vi "ContextHelp_Memory.vi"(0 "PopUpTaskEvent":T1, 1 "State":bool, 5 "error in (no error)":errorcluster, 6 "Actio(GetStatus)n":T2(ring)=enum."GetStatus") -> (14 "PopUpTaskEventOut":T1, 15 "Open":bool, 16 "DialogCaller":bool, 17 "DialogRef":refnum<vi>, 18 "ToolHelp":bool, 19 "error out":errorcluster)   [LabVIEW 2016]
uses:
  <resource>/Framework/Providers/Open_GDS/UML/ContextHelp/ContextHelp_EventType.ctl
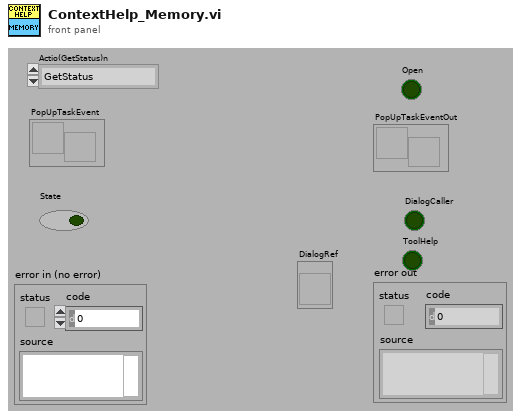
[diagram p1: front panel]
types:
  T1 = typedef "ContextHelp_EventType.ctl" = refnum<user-event>
  T2 = enum16{"SetPopUpEventTask", "GetStatus", "SetOpenState", "SetDialogCaller", "SetToolHelp"}
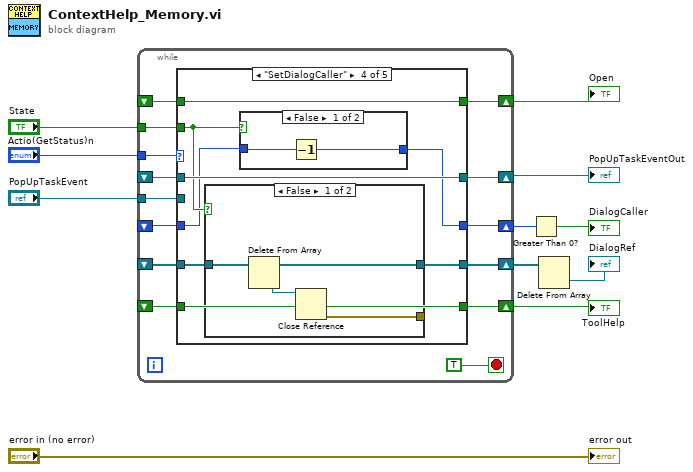
[diagram p0: block diagram]
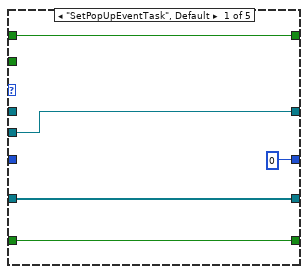
[diagram p2: hidden frame]
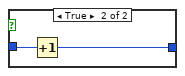
[diagram p5: hidden frame]
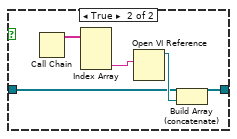
[diagram p6: hidden frame]
diagram:
  n1 = while {
    tunnel: "Actio(GetStatus)n" -> [w25]
    shift-right: [w23] -> w9
    shift-left: _ -> [w24]
    tunnel: "State" -> [w22]
    shift-right: [w21] -> w6
    shift-left: _ -> [w19]
    tunnel: "PopUpTaskEvent" -> [w20]
    shift-right: [w17] -> w4
    shift-left: _ -> [w16]
    shift-right: [w15] -> w2
    shift-left: _ -> [w14]
    shift-right: [w13] -> w5
    shift-left: _ -> [w12]
    stop <- TRUE stop-if-true
    n2 = case shown="\"SetDialogCaller\"" w25 {
      tunnel: w24 -> [w30 _ w36 w47 w66]
      tunnel: [w30 w35 w36 w47 w66] -> w23
      tunnel: w22 -> [_ w35 w37 w43 _]
      tunnel: [w29 w34 w40 w48 w65] -> w21
      tunnel: w20 -> [w29 _ _ _ _]
      tunnel: w19 -> [_ w34 w40 w48 w65]
      tunnel: [0 w33 w39 w41 w64] -> w17
      tunnel: w16 -> [_ w33 w39 w42 w64]
      tunnel: [w28 w32 w38 w46 w63] -> w15
      tunnel: w14 -> [w28 w32 w38 w45 w63]
      tunnel: [w27 w31 w37 w44 w62] -> w13
      tunnel: w12 -> [w27 w31 _ w44 w62]
      frame "SetPopUpEventTask", Default {
      }
      frame "SetOpenState" {
      }
      frame "SetToolHelp" {
      }
      frame "SetDialogCaller" {
        n3 = case shown="False" w43 {
          tunnel: [w54 w58] -> w46
          tunnel: w45 -> [w55 w57]
          tunnel: [w53 _] -> _
          frame False {
            n4 = Delete From Array(array=w55) -> (deleted portion=w56:refnum<vi>, array with subset deleted=w54:refnum<vi>[])  [unwired: 2 in]
            n5 = Close Reference(reference=w56) -> (error out=w53:errorcluster)  [unwired: 1 in]
          }
          frame True {
            n6 = Call Chain() -> (call chain=w61:string[])
            n7 = Index Array(array=w61) -> (element #3=w60:string)  [unwired: 3 in, 2 out]
            n8 = Open VI Reference(vi path=w60) -> (vi reference=w59:refnum<vi>)  [unwired: 1 in, 5 out]
            n9 = Build Array (concatenate)(w57, w59) -> (w58:refnum<vi>[])
          }
        }
        n10 = case shown="False" w43 {
          tunnel: w42 -> [w50 w52]
          tunnel: [w49 w51] -> w41
          frame False {
            n11 = Decrement(x=w50) -> (x-1=w49:i32)
          }
          frame True {
            n12 = Increment(x=w52) -> (x+1=w51:i32)
          }
        }
      }
      frame "GetStatus" {
      }
    }
  }
  "Open" <- w9
  "PopUpTaskEventOut" <- w6
  "ToolHelp" <- w5
  n13 = Greater Than 0?(x=w4) -> (x > 0?=→"DialogCaller":bool)
  n14 = Delete From Array(array=w2) -> (deleted portion=→"DialogRef":refnum<vi>)  [unwired: 2 in, 1 out]
  "error out" <- "error in (no error)"
